vi "niDTS GNSS GPS Rx RF Test Configure.vi"(0 "Template Tx Test Handle in":T3, 7 "Parameters":T1 {"External Attenuation (dB)" format="%.1g"; "Power (dBm)" format="%.1g"}, 9 "ResultsIndex":u8=1, 11 "error in (no error)":errorcluster) -> (4 "Template Tx Test Handle out":T3, 15 "error out":errorcluster)   [LabVIEW 2014, in "niDTS GNSS.lvlib"]
uses:
  niDTS GNSS.lvlib
  RF Test/Includes/niDTS GNSS RF Test INC Handle.ctl
  RF Test/Objects/BASE_class/niDTS GNSS RF Test.lvclass
  Includes/niDTS GNSS GPS Rx RF Test INC Parameters.ctl
  Includes/niDTS GNSS GPS Rx RF Test INC Channel.ctl
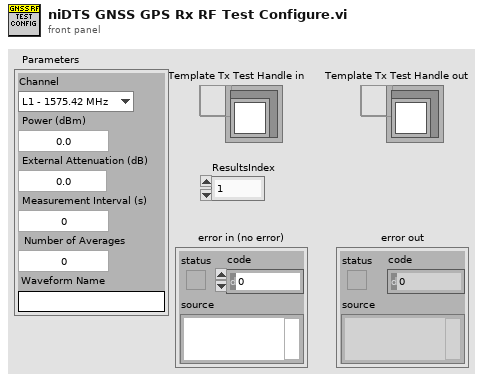
[diagram p1: front panel]
types:
  T1 = typedef "niDTS GNSS.lvlib/niDTS GNSS GPS Rx RF Test INC Parameters.ctl" = cluster{"Channel":T2, "Power (dBm)":dbl, "External Attenuation (dB)":dbl, "Measurement Interval (s)":dbl, "Number of Averages":i32, "Waveform Name":string}
  T2 = typedef "niDTS GNSS.lvlib/niDTS GNSS GPS Rx RF Test INC Channel.ctl" = enum16{"L1 - 1575.42 MHz", "L2 - 1227.60 MHz", "L5 - 1176.45 MHz"}
  T3 = typedef "niDTS GNSS.lvlib/niDTS GNSS RF Test INC Handle.ctl" = refnum<data-value>
  T4 = typedef "niDTS GNSS.lvlib/niDTS GNSS RF Test INC Parameters.ctl" = cluster{"GNSS Standard":enum16{"GPS", "GLONASS", "Galileo", "Beidou"}, "Frequency (Hz)":dbl, "Auto Level":bool, "Power (dBm)":dbl, "External Attenuation (dB)":dbl, "Measurement Interval (s)":dbl, "Pattern":enum16{"0", "1", "01", "00001111", "PN9"}, "Enable Averaging":bool, "Type Of Averaging":enum16{"MEAN", "MAX", "MIN", "MAXMIN"}, "Number of Averages":i32, "Waveform Name":string, "Enable Traces":bool}
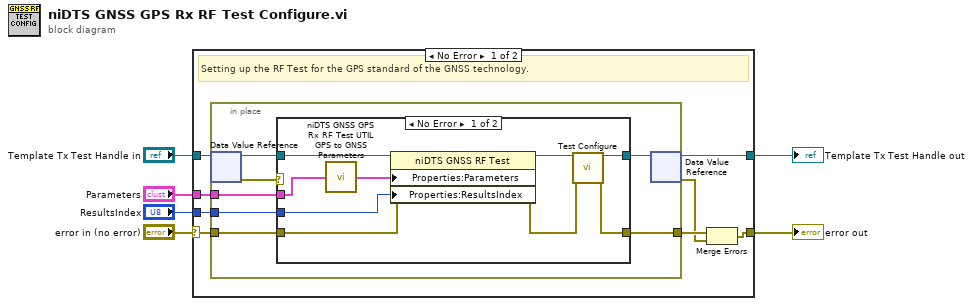
[diagram p0: block diagram]
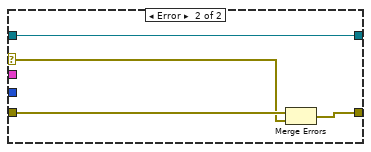
[diagram p2: hidden frame]
diagram:
  n1 = case shown="No Error" "error in (no error)" {
    selector: "error in (no error)" -> [w10 w36]
    tunnel: "Parameters" -> [w14 _]
    tunnel: "Template Tx Test Handle in" -> [w13 w35]
    tunnel: [w12 w35] -> w4
    tunnel: [w9 w36] -> w3
    tunnel: "ResultsIndex" -> [w11 _]
    frame No Error {
      # "Setting up the RF Test for the GPS standard of the GNSS technology."
      n2 = in-place {
        in-place-border: w10 -> [w18]
        in-place-border: [w17] -> w8
        in-place-border: w14 -> [w16]
        in-place-border: w11 -> [w15]
        n3 = in-place-dvr #1(w13) -> (w20:refnum<class "niDTS GNSS RF Test.lvclass">, w21:errorcluster)
        n4 = case shown="No Error" w21 {
          selector: w21 -> [_ w32]
          tunnel: w20 -> [w30 w34]
          tunnel: [w26 w34] -> w19
          tunnel: w18 -> [w29 w33]
          tunnel: [w27 w31] -> w17
          tunnel: w16 -> [w23 _]
          tunnel: w15 -> [w24 _]
          frame No Error {
            n5 = call "niDTS GNSS GPS Rx RF Test UTIL GPS to GNSS Parameters.vi"("Parameters IN"=w23) -> ("Parameters OUT"=w22:T4)
            n6 = property class="niDTS GNSS RF Test"(reference=w30, error in=w29, "Properties:Parameters"=w22, "Properties:ResultsIndex"=w24) -> (reference out=w25:refnum<class "niDTS GNSS RF Test.lvclass">, error out=w28:errorcluster)
            n7 = call-dynamic "Test Configure.vi"("Template RF Test in"=w25, "error in (no error)"=w28) -> ("Template RF Test out"=w26:refnum<class "niDTS GNSS RF Test.lvclass">, "error out"=w27:errorcluster)  [unwired: 12 in]
          }
          frame Error {
            n8 = Merge Errors(w33, w32) -> (w31:errorcluster)
          }
        }
        n9 = in-place-dvr #1(w19) -> (w12:T3, w7:errorcluster)
      }
      n10 = Merge Errors(w8, w7) -> (w9:errorcluster)
    }
    frame Error {
    }
  }
  "Template Tx Test Handle out" <- w4
  "error out" <- w3
